vi "Stop Saving.vi"(8 "error in (no error)":errorcluster, 11 "Digital Acquisition in":refnum<class "Digital Acquisition.lvclass">) -> (0 "error out":errorcluster, 3 "Digital Acquisition out":refnum<class "Digital Acquisition.lvclass">)   [LabVIEW 2020, in "Digital Acquisition.lvlib" / "Digital Acquisition.lvclass"]
uses:
  Digital Acquisition.lvclass
  C:/Program Files (x86)/National Instruments/LabVIEW 2020/vi.lib/ActorFramework/Actor/Actor.lvclass
  <vilib>/ActorFramework/Actor/Actor.lvclass/Actor.ctl
  <vilib>/ActorFramework/Message Enqueuer/Message Enqueuer.lvclass/Message Enqueuer.ctl
  Digital Acquisition.lvclass/Digital Acquisition.ctl
  Digital Acquisition Messages/Update File Name Indicator Msg/Update File Name Indicator Msg.lvclass/Update File Name Indicator Msg.ctl
  <vilib>/ActorFramework/Message Enqueuer/Init from Existing Queue.vi
  <vilib>/ActorFramework/Message Enqueuer/Enqueue.vi
  <vilib>/ActorFramework/Stop Msg/Stop Msg.lvclass
  C:/Program Files (x86)/National Instruments/LabVIEW 2020/vi.lib/ActorFramework/Message/Message.lvclass
  Digital Acquisition Messages/Update File Name Indicator Msg/Update File Name Indicator Msg.lvclass
  <vilib>/ActorFramework/Message Priority Queue/Priority Enqueue.vi
  <vilib>/ActorFramework/Message Enqueuer/Message Enqueuer.lvclass
  <vilib>/ActorFramework/Actor/Actor.lvclass
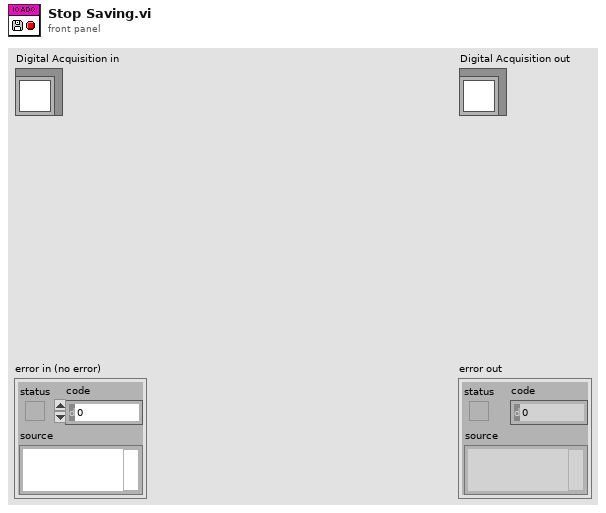
[diagram p1: front panel]
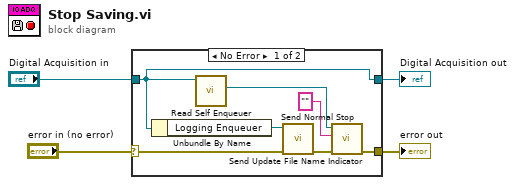
[diagram p0: block diagram]
diagram:
  n1 = case shown="No Error" "error in (no error)" {
    selector: "error in (no error)" -> [w11 w13]
    tunnel: [w5 w13] -> w3
    tunnel: [w9 w12] -> w1
    tunnel: "Digital Acquisition in" -> [w9 w12]
    frame No Error {
      n2 = Unbundle By Name(w9) -> ("Logging Enqueuer"=w10:refnum<class "Message Enqueuer.lvclass">)
      n3 = call <vilib>:"Read Self Enqueuer.vi"("Actor"=w9) -> ("Self Enqueuer"=w8:refnum<class "Message Enqueuer.lvclass">)  [unwired: 10 in]
      n4 = call <vilib>:"Send Normal Stop.vi"("error in (no error)"=w11, "Message Enqueuer"=w10) -> ("error out"=w6:errorcluster)  [unwired: 9 in]
      n5 = call "Send Update File Name Indicator.vi"("error in (no error)"=w6, "File Name"="", "Message Enqueuer"=w8) -> ("error out"=w5:errorcluster)  [unwired: 7 in, 1 out]
    }
    frame Error {
    }
  }
  "error out" <- w3
  "Digital Acquisition out" <- w1
